vi "Get All Project Strings from Definition.vi"(4 "error in":errorcluster) -> (0 "error out":errorcluster, 3 "Project Strings":T1[](array[typedef]))   [LabVIEW 2025]
doc: "This VI generates an array of clusters that contain the name of each Project in the <i>Test Project Definition.xml</i> file, followed by all strings defined for each Project (i.e. all strings of each VI, Cluster and Class which is part of the project).\n\nStrings that are added to the project due to a member element receive an identifier (e.g. [source VI]).\n\nThis information is used to assert correct functioning of <b>Export Strings.vi</b>"
uses:
  Element Strings--cluster.ctl
  Project Definition--cluster.ctl
  <userlib>/_OpenG.lib/file/file.llb/Strip Path - Arrays__ogtk.vi
  <userlib>/_OpenG.lib/file/file.llb/openg_file.lvlib
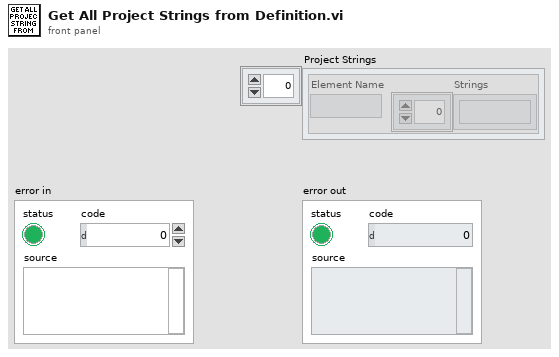
[diagram p1: front panel]
types:
  T1 = typedef "Element Strings--cluster.ctl" = cluster{"Element Name":string, "Strings":string[]}
  T2 = typedef "Project Definition--cluster.ctl" = cluster{"Name":string, "Description":string, "Elements":path[]}
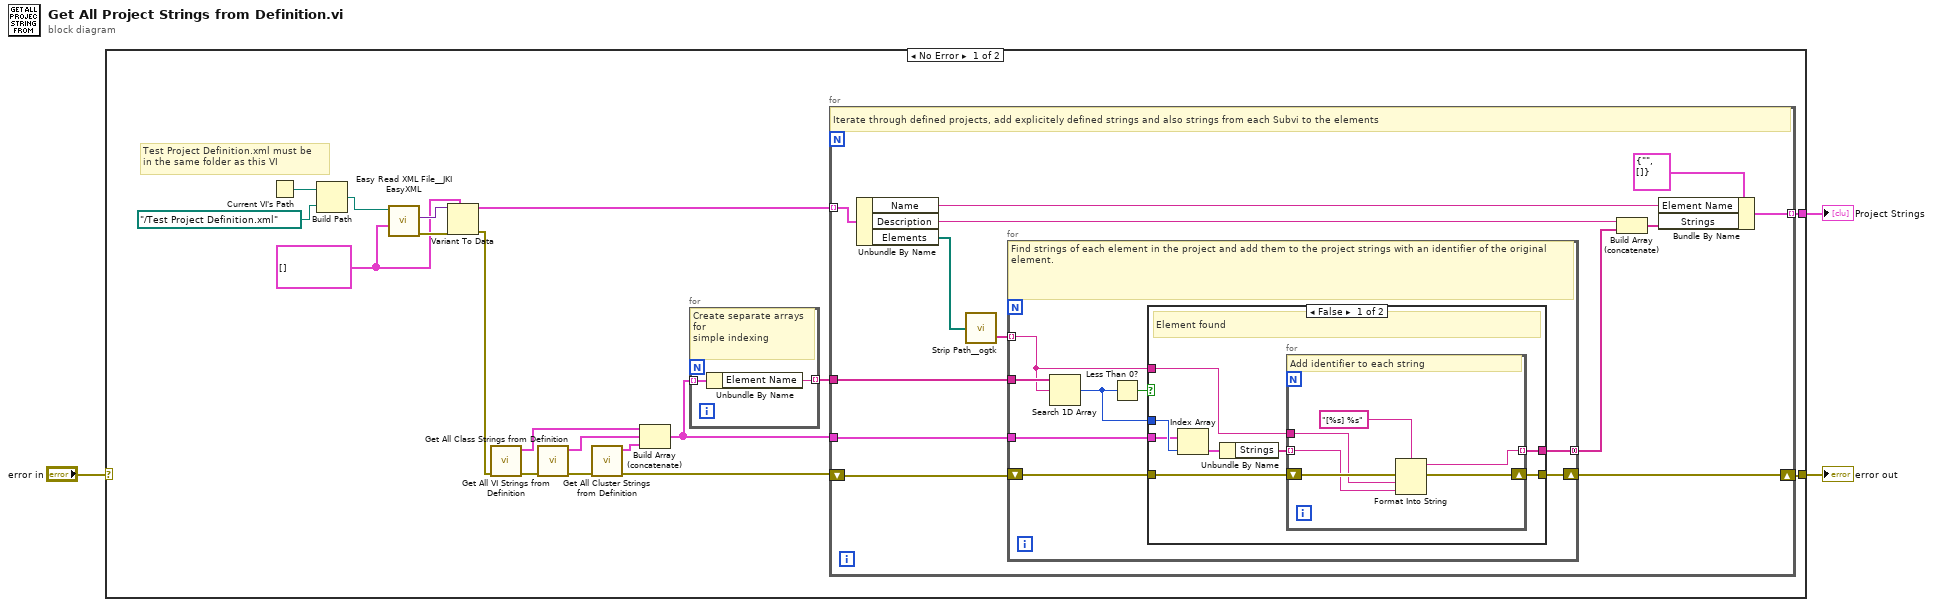
[diagram p0: block diagram]
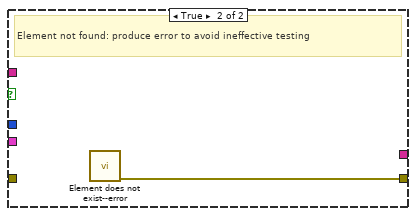
[diagram p2: hidden frame]
diagram:
  n1 = case shown="No Error" "error in" {
    selector: "error in" -> [_ w60]
    tunnel: [w14 _] -> w3
    tunnel: [w8 w60] -> w2
    frame No Error {
      w16 = T2[] [] ("Array")
      # "Test Project Definition.xml must be\nin the same folder as this VI"
      n2 = Current VI's Path() -> (path=w21:path)
      n3 = Build Path(base path=w21, name or relative path=path "../Test Project Definition.xml") -> (appended path=w19:path)
      n4 = call <vilib>:"Easy Read XML File__JKI EasyXML.vi"("LabVIEW Data (Type)"=w16, "XML File Path"=w19) -> ("error out"=w17:errorcluster, "LabVIEW Data"=w18:variant)  [unwired: 7 in, 1 out]
      n5 = Variant To Data(error in=w17, type=w16, Variant=w18) -> (data=w15:T2[], error out=w13:errorcluster)
      n6 = call "Get All VI Strings from Definition.vi"("error in"=w13) -> ("error out"=w12:errorcluster, "VI Strings"=w11:T1[])  [unwired: 5 in]
      n7 = call "Get All Class Strings from Definition.vi"("error in"=w12) -> ("error out"=w6:errorcluster, "VI Strings"=w10:T1[])  [unwired: 5 in]
      n8 = call "Get All Cluster Strings from Definition.vi"("error in"=w6) -> ("error out"=w5:errorcluster, "Cluster Strings"=w4:T1[])  [unwired: 5 in]
      n9 = Build Array (concatenate)(w11, w10, w4) -> (w7:T1[])
      n10 = for {
        tunnel: w7 -> [w23] mode=indexing
        tunnel: [w22] -> w9 mode=indexing
        # "Create separate arrays for\nsimple indexing"
        n11 = Unbundle By Name(w23) -> ("Element Name"=w22:string)
      }
      n12 = for {
        tunnel: w15 -> [w35] mode=indexing
        tunnel: [w33] -> w14 mode=indexing
        shift-right: [w24] -> w8
        shift-left: w5 -> [w25]
        tunnel: w9 -> [w28]
        tunnel: w7 -> [w26]
        # "Iterate through defined projects, add explicitely defined strings and also strings from each Subvi to the elements"
        n13 = Unbundle By Name(w35) -> ("Name"=w34:string, "Description"=w32:string, "Elements"=w30:path[])
        n14 = call-poly <userlib>:"Strip Path__ogtk.vi"("path"=w30) -> ("name"=w29:string[])  [unwired: 1 out]
        n15 = for {
          tunnel: w29 -> [w37] mode=indexing
          tunnel: w28 -> [w44]
          tunnel: [w43] -> w27 mode=concatenating
          tunnel: w26 -> [w40]
          shift-right: [w38] -> w24
          shift-left: w25 -> [w39]
          # "Find strings of each element in the project and add them to the project strings with an identifier of the original element."
          n16 = Search 1D Array(1D array=w44, element=w37) -> (index of element=w42:i32)  [unwired: 1 in]
          n17 = Less Than 0?(x=w42) -> (x < 0?=w41:bool)
          n18 = case shown="False" w41 {
            tunnel: w42 -> [w52 _]
            tunnel: w40 -> [w51 _]
            tunnel: [w46 _] -> w43
            tunnel: w39 -> [w48 _]
            tunnel: [w45 w59] -> w38
            tunnel: w37 -> [w47 _]
            frame False {
              # "Element found"
              n19 = Index Array(array=w51, index=w52) -> (element=w50:T1)
              n20 = Unbundle By Name(w50) -> ("Strings"=w49:string[])
              n21 = for {
                tunnel: w49 -> [w55] mode=indexing
                shift-right: [w56] -> w45
                shift-left: w48 -> [w57]
                tunnel: w47 -> [w54]
                tunnel: [w53] -> w46 mode=indexing
                # "Add identifier to each string"
                n22 = Format Into String(format string="[%s] %s", error in=w57, w54, w55) -> (resulting string=w53:string, error out=w56:errorcluster)  [unwired: 1 in]
              }
            }
            frame True {
              # "Element not found: produce error to avoid ineffective testing"
              n23 = call "Element does not exist--error.vi"() -> ("error out"=w59:errorcluster)  [unwired: 7 in]
            }
          }
        }
        n24 = Build Array (concatenate)(w32, w27) -> (w31:string[])
        n25 = Bundle By Name(cluster=T1 {"Element Name"="", "Strings"=[]} ("VI Strings"), "Element Name"=w34, "Strings"=w31) -> (w33:T1)
      }
    }
    frame Error {
      # "Pass error without further actions"
    }
  }
  "Project Strings" <- w3
  "error out" <- w2
